vi "sensor value to int.vi"(8 "error in (no error)":errorcluster, 10 "value_out":i32, 11 "h":u64) -> (0 "error out":errorcluster, 2 "value_out out":i32, 3 "function return":u32(ring))   [LabVIEW 2023, in "uhd.lvlib"]
doc: "UHD_API uhd_error uhd_sensor_value_to_int(uhd_sensor_value_handle h, int* value_out);"
uses:
  <userlib>/uhd/uhd.lvlib
  <userlib>/uhd/uhd.dll
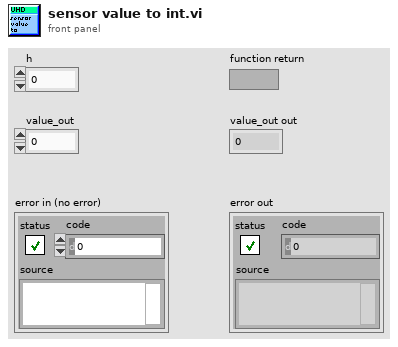
[diagram p1: front panel]
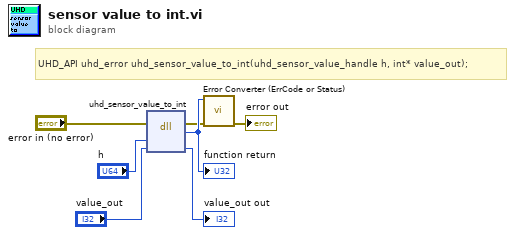
[diagram p0: block diagram]
diagram:
  # "UHD_API uhd_error uhd_sensor_value_to_int(uhd_sensor_value_handle h, int* value_out);"
  n1 = dll-call lib="C:/Program Files/National Instruments/LabVIEW 2023/user.lib/uhd/uhd.*" fn="uhd_sensor_value_to_int"(error in="error in (no error)", "h"="h", "value_out"="value_out") -> (error out=w2:errorcluster, w7:u32, "value_out"=→"value_out out":i32)  [unwired: 3 in, 1 out]
  "function return" <- w7
  n2 = call <userlib>:"Error Converter (ErrCode or Status).vi"("error in (no error)"=w2, "error code"=w7) -> ("error out"=→"error out":errorcluster)  [unwired: 9 in]
